vi "ToRawCommands_RT.vi"(1 "Macro Info 2D":T1(array[cluster])=[[{"Duration (s)"=0.001, "Instruction Description"="Initial state", "Input Bits"=[FALSE, FALSE, FALSE, FALSE, FALSE, FALSE, FALSE, FALSE, FALSE, FALSE, FALSE, FALSE, FALSE, FALSE, FALSE, FALSE], "Output Bits"=[FALSE, FALSE, FALSE, FALSE, FALSE, FALSE, FALSE, FALSE, FALSE, FALSE, FALSE, FALSE, FALSE, FALSE, FALSE, FALSE, FALSE, FALSE, FALSE, FALSE, FALSE, FALSE, FALSE, FALSE, FALSE, FALSE, FALSE, FALSE, FALSE, FALSE, FALSE, FALSE, FALSE, FALSE, FALSE, FALSE, FALSE, FALSE], "DAC levels (V)"=[0.0, 0.0, 0.0, 0.0, 0.0, 0.0, 0.0, 0.0, 0.0, 0.0, 0.0, 0.0, 0.0, 0.0, 0.0, 0.0], "Steps"=2, "Changes"=[TRUE, TRUE]}, {"Duration (s)"=0.001, "Instruction Description"="Ramp up", "Input Bits"=[FALSE, FALSE, FALSE, FALSE, FALSE, FALSE, FALSE, FALSE, FALSE, FALSE, FALSE, FALSE, FALSE, FALSE, FALSE, FALSE], "Output Bits"=[TRUE, FALSE, FALSE, FALSE, FALSE, FALSE, FALSE, FALSE, FALSE, FALSE, FALSE, FALSE, FALSE, FALSE, FALSE, FALSE, FALSE, FALSE, FALSE, FALSE, FALSE, FALSE, FALSE, FALSE, FALSE, FALSE, FALSE, FALSE, FALSE, FALSE, FALSE, FALSE, FALSE, FALSE, FALSE, FALSE, FALSE, FALSE], "DAC levels (V)"=[5.0, 0.0, 0.0, 0.0, 0.0, 0.0, 0.0, 0.0, 0.0, 0.0, 0.0, 0.0, 0.0, 0.0, 0.0, 5.0], "Steps"=10, "Changes"=[TRUE, TRUE]}, {"Duration (s)"=0.001, "Instruction Description"="Zero all", "Input Bits"=[FALSE, FALSE, FALSE, FALSE, FALSE, FALSE, FALSE, FALSE, FALSE, FALSE, FALSE, FALSE, FALSE, FALSE, FALSE, FALSE], "Output Bits"=[FALSE, FALSE, FALSE, FALSE, FALSE, FALSE, FALSE, FALSE, FALSE, FALSE, FALSE, FALSE, FALSE, FALSE, FALSE, FALSE, FALSE, FALSE, FALSE, FALSE, FALSE, FALSE, FALSE, FALSE, FALSE, FALSE, FALSE, FALSE, FALSE, FALSE, FALSE, FALSE, FALSE, FALSE, FALSE, FALSE, FALSE, FALSE], "DAC levels (V)"=[0.0, 0.0, 0.0, 0.0, 0.0, 0.0, 0.0, 0.0, 0.0, 0.0, 0.0, 0.0, 0.0, 0.0, 0.0, 0.0], "Steps"=2, "Changes"=[TRUE, TRUE]}]], 2 "# AO cards":u8=2) -> (0 "RAW cluster":cluster{i16[][]}[][](array[cluster])=[[{[[0, 0, 0, 0, 0, 0, 0, 0, 0, 0, 0, 0, 0, 0, 0, 0], [0, 0, 0, 0, 0, 0, 0, 0, 0, 0, 0, 0, 0, 0, 0, 0]]}, {[[0, 0, 0, 0, 0, 0, 0, 0, 1820, 0, 0, 0, 0, 0, 0, 0, 3641, 0, 0, 0, 0, 0, 0, 0, 5461, 0, 0, 0, 0, 0, 0, 0, 7282, 0, 0, 0, 0, 0, 0, 0, 9102, 0, 0, 0, 0, 0, 0, 0, 10923, 0, 0, 0, 0, 0, 0, 0, 12743, 0, 0, 0, 0, 0, 0, 0, 14564, 0, 0, 0, 0, 0, 0, 0, 16384, 0, 0, 0, 0, 0, 0, 0], [0, 0, 0, 0, 0, 0, 0, 0, 0, 0, 0, 0, 0, 0, 0, 1820, 0, 0, 0, 0, 0, 0, 0, 3641, 0, 0, 0, 0, 0, 0, 0, 5461, 0, 0, 0, 0, 0, 0, 0, 7282, 0, 0, 0, 0, 0, 0, 0, 9102, 0, 0, 0, 0, 0, 0, 0, 10923, 0, 0, 0, 0, 0, 0, 0, 12743, 0, 0, 0, 0, 0, 0, 0, 14564, 0, 0, 0, 0, 0, 0, 0, 16384]]}, {[[16384, 0, 0, 0, 0, 0, 0, 0, 0, 0, 0, 0, 0, 0, 0, 0], [0, 0, 0, 0, 0, 0, 0, 16384, 0, 0, 0, 0, 0, 0, 0, 0]]}]])   [LabVIEW 2018]
uses:
  <vilib>/Analysis/1siggen.llb/Ramp Pattern by Samples.vi
  <vilib>/Analysis/NI_AALBase.lvlib
panel:
  out "Last levels (V)":dbl[](array[numeric])
  out "Instruction":i32=2
  out "Action":i32
  # "RAW cmds: \n  Actions\n  |- Instructions\n      |-  AO cards\n           |-  integer arrays"
  # "Action"
  # "Instruction"
  # "AO card"
  # "RAWindex"
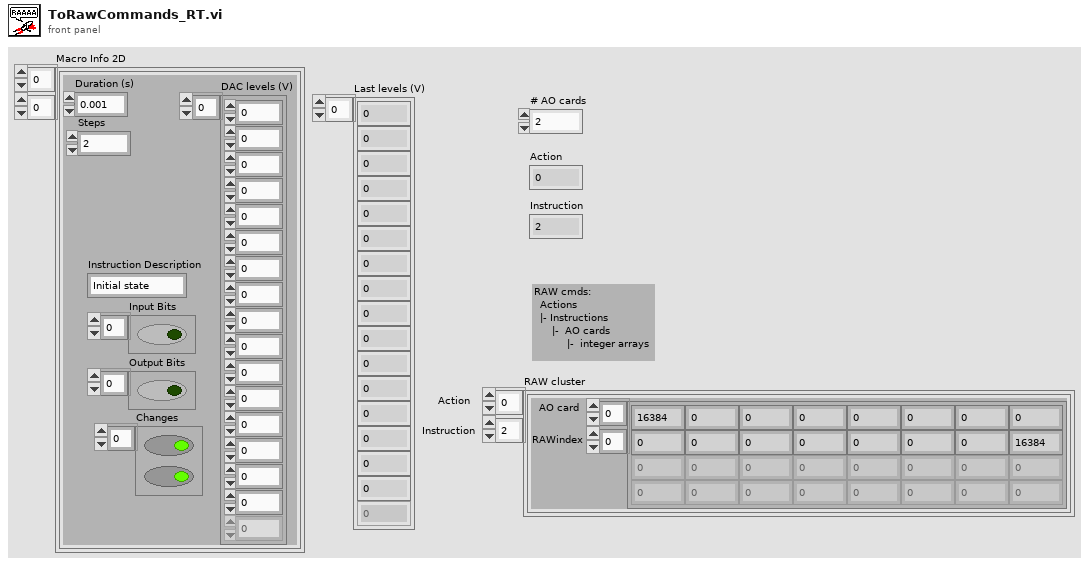
[diagram p1: front panel]
types:
  T1 = cluster{"Duration (s)":dbl, "Instruction Description":string, "Input Bits":bool[], "Output Bits":bool[], "DAC levels (V)":dbl[], "Steps":i32, "Changes":bool[]}[][]
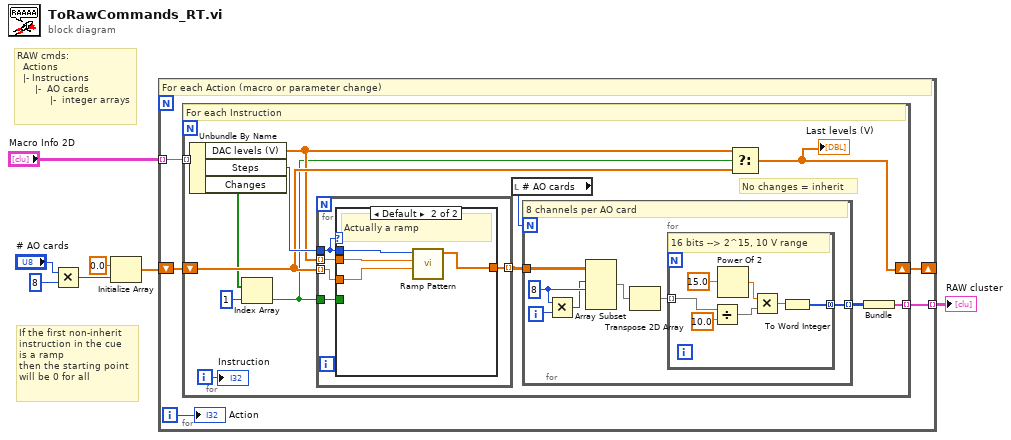
[diagram p0: block diagram]
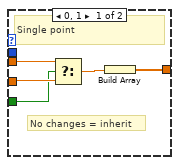
[diagram p2: hidden frame]
diagram:
  # "If the first non-inherit\ninstruction in the cue\nis a ramp\nthen the starting point\nwill be 0 for all"
  # "RAW cmds:\n  Actions\n  |- Instructions\n      |-  AO cards\n           |-  integer arrays"
  n1 = Multiply(x="# AO cards", y=8) -> (x*y=w2:i32)
  n2 = Initialize Array(0.0 ("element"), w2) -> (w6:dbl[])
  n3 = for {
    tunnel: "Macro Info 2D" -> [w10] mode=indexing
    shift-right: [w11] -> _
    shift-left: w6 -> [w12]
    tunnel: [w9] -> w1 mode=indexing
    i -> [w8]
    # "For each Action (macro or parameter change)"
    n4 = for {
      tunnel: w10 -> [w25] mode=indexing
      shift-right: [w18] -> w11
      shift-left: w12 -> [w17]
      tunnel: [w21] -> w9 mode=indexing
      i -> [w19]
      # "No changes = inherit"
      # "For each Instruction"
      n5 = Unbundle By Name(w25) -> ("DAC levels (V)"=w16:dbl[], "Steps"=w24:i32, "Changes"=w15:bool[])
      n6 = Index Array(array=w15, index=1) -> (element=w13:bool)
      n7 = for {
        tunnel: w17 -> [w44] mode=indexing
        tunnel: w16 -> [w43] mode=indexing
        tunnel: w24 -> [w41]
        tunnel: [w42] -> w23 mode=indexing
        tunnel: w13 -> [w40]
        n8 = case shown="Default" w41 {
          tunnel: w44 -> [w46 w53]
          tunnel: w43 -> [w47 w52]
          tunnel: w41 -> [_ w51]
          tunnel: [w49 w50] -> w42
          tunnel: w40 -> [w45 _]
          frame 0, 1 {
            # "No changes = inherit"
            # "Single point"
            n9 = Select(t=w47, s=w45, f=w46) -> (s? t:f=w48:dbl)
            n10 = Build Array(w48) -> (w49:dbl[])
          }
          frame Default {
            # "Actually a ramp"
            n11 = call-poly <vilib>:"Ramp Pattern.vi"("start"=w53, "end"=w52, "samples"=w51) -> ("Ramp Pattern"=w50:dbl[])  [unwired: 7 in, 1 out]
          }
        }
      }
      n12 = local read "# AO cards"() -> (w22:u8)
      n13 = for {
        N: w22 -> [_]
        tunnel: w23 -> [w32]
        tunnel: [w27] -> w20 mode=indexing
        i -> [w31]
        w30 = 8 ("length")
        # "8 channels per AO card"
        n14 = Multiply(x=w30, y=w31) -> (x*y=w29:i32)
        n15 = Array Subset(array=w32, index (row)=w29, length (row)=w30) -> (w26:dbl[][])  [unwired: 2 in]
        n16 = Transpose 2D Array(2D array=w26) -> (transposed array=w28:dbl[][])
        n17 = for {
          tunnel: w28 -> [w34] mode=indexing
          tunnel: [w33] -> w27 mode=concatenating
          # "16 bits --> 2^15, 10 V range"
          n18 = Divide(x=w34, y=10.0) -> (x/y=w39:dbl[])
          n19 = Power Of 2(x=15.0) -> (2^x=w38:dbl)
          n20 = Multiply(x=w38, y=w39) -> (x*y=w37:dbl[])
          n21 = To Word Integer(number=w37) -> (16bit integer=w33:i16[])
        }
      }
      n22 = Select(t=w16, s=w13, f=w17) -> (s? t:f=w18:dbl[])
      "Last levels (V)" <- w18
      n23 = Bundle(w20) -> (w21:cluster{i16[][]})  [unwired: 1 in]
      "Instruction" <- w19
    }
    "Action" <- w8
  }
  "RAW cluster" <- w1
